vi "MBytes to Bytes.vi"(7 "MBytes":dbl) -> (4 "kBytes":u32, 8 "Bytes":u32)   [LabVIEW 2013]
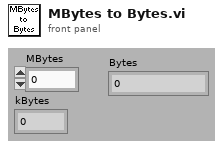
[diagram p1: front panel]
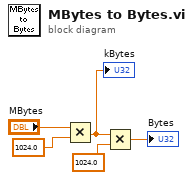
[diagram p0: block diagram]
diagram:
  n1 = Multiply(x="MBytes", y=1024.0) -> (x*y=w3:dbl)
  "kBytes" <- w3
  n2 = Multiply(x=w3, y=1024.0) -> (x*y=→"Bytes":dbl)
